vi "Actor Core.vi"(8 "error in":errorcluster, 11 "Manual UI in":refnum<class "Manual UI.lvclass">) -> (0 "error out":errorcluster, 3 "Actor out":refnum<class "Actor.lvclass">)   [LabVIEW 2019, in "Manual UI.lvlib" / "Manual UI.lvclass"]
doc: "The user interface for the main gui panel.\nThis UI manages splitter positions and instrument panels."
uses:
  Project/Manual UI.lvclass
  C:/Users/Public/Documents/Development/builds/Engine/Engine.lvlibp/Project/Engine.lvclass
  builds/Engine/Actor Framework.lvlibp/1abvi3w/vi.lib/ActorFramework/Actor/Actor.lvclass
  Project/Manual UI.lvclass/Manual UI.ctl
  Manual UI Messages/Change Active Instrument Msg/Change Active Instrument Msg.lvclass/Change Active Instrument Msg.ctl
  Accessors/Write instrSplitters.vi
  Accessors/Write instrPanels.vi
  builds/Engine/Engine.lvlibp/Accessors/Write VI_Ref.vi
  builds/Engine/Engine.lvlibp/Accessors/Read Self Q.vi
  builds/Engine/Actor Framework.lvlibp/1abvi3w/vi.lib/ActorFramework/Message Enqueuer/Enqueue.vi
  builds/Engine/Actor Framework.lvlibp/1abvi3w/vi.lib/ActorFramework/Message Enqueuer/Message Enqueuer.lvclass
  Manual UI Messages/Change Active Instrument Msg/Change Active Instrument Msg.lvclass
  Manual UI Messages/Close Instruments Msg/Close Instruments Msg.lvclass
  Manual UI Messages/Launch Instruments Msg/Launch Instruments Msg.lvclass
  builds/Base Software/Panels/Prime Panel.lvlibp/Project/Prime Panel.lvclass
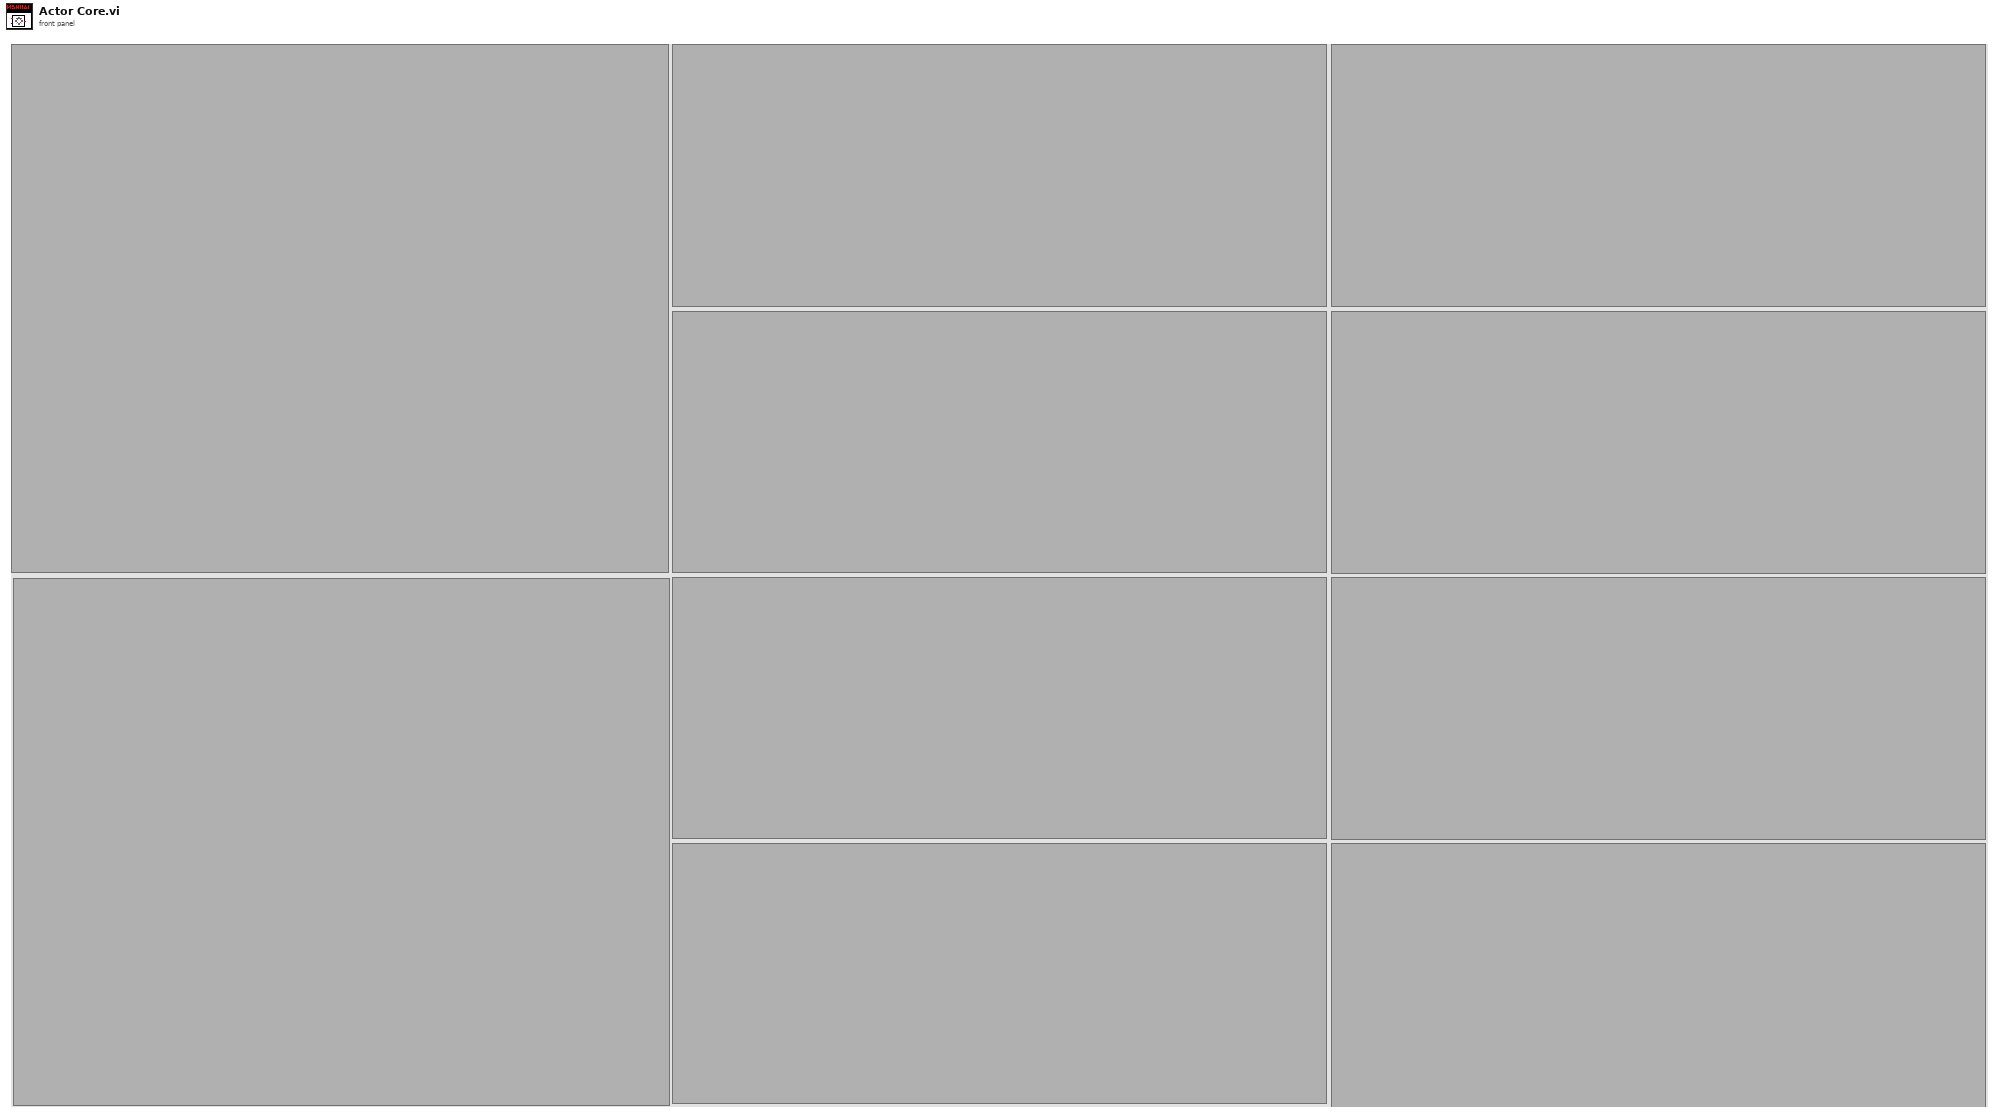
[diagram p1: front panel]
types:
  T1 = cluster{"Pnl Actor":refnum<event-registration>, "Event Registration Refnum":refnum<event-registration>}
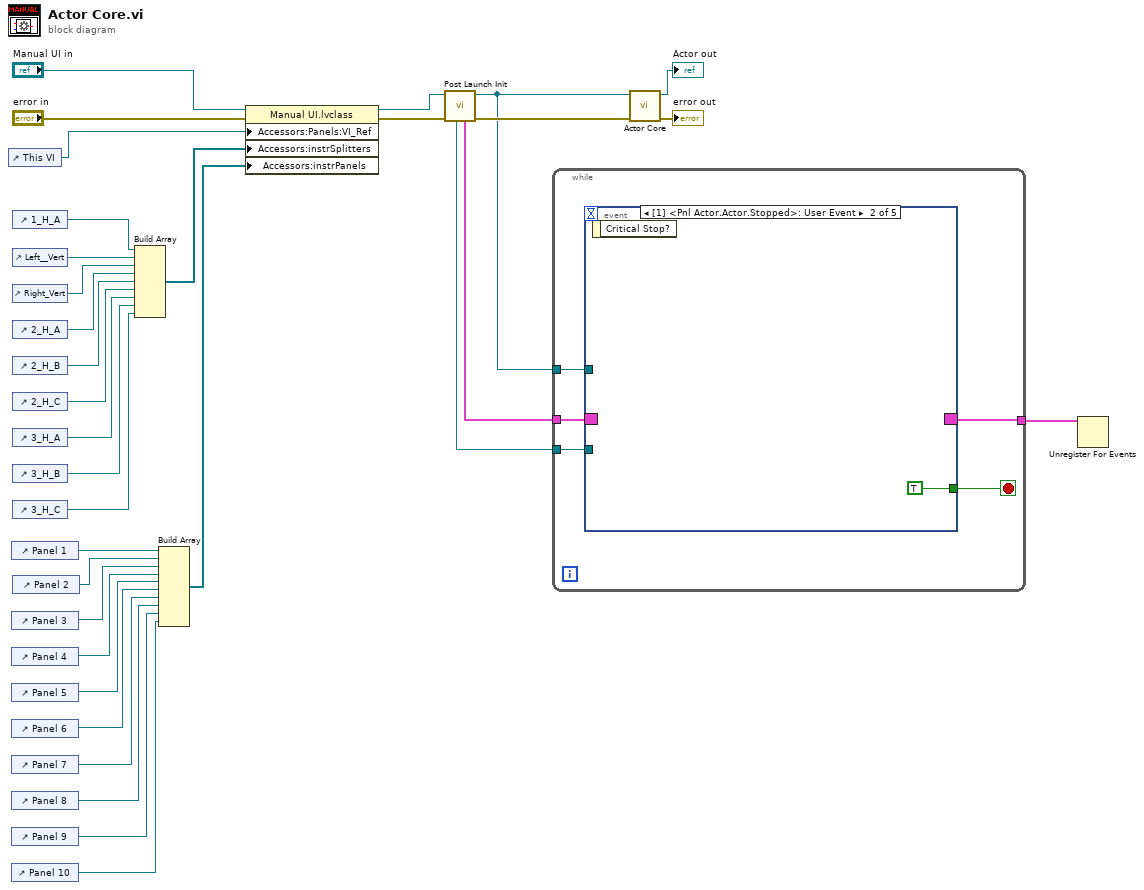
[diagram p0: block diagram]
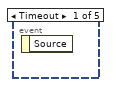
[diagram p2: hidden frame]
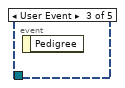
[diagram p3: hidden frame]
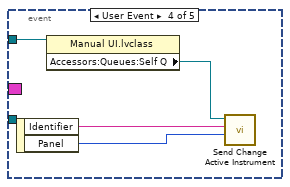
[diagram p4: hidden frame]
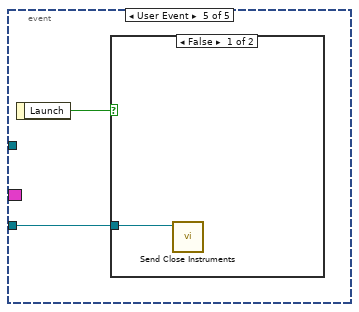
[diagram p5: hidden frame]
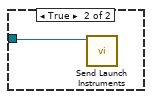
[diagram p6: hidden frame]
diagram:
  n1 = control-ref of="This VI"() -> (w7:refnum<vi>)
  n2 = control-ref of="Panel 1"() -> (w21:refnum<vi>)
  n3 = control-ref of="Panel 3"() -> (w20:refnum<vi>)
  n4 = control-ref of="Panel 4"() -> (w19:refnum<vi>)
  n5 = control-ref of="Panel 5"() -> (w18:refnum<vi>)
  n6 = control-ref of="Panel 6"() -> (w17:refnum<vi>)
  n7 = control-ref of="Panel 7"() -> (w16:refnum<vi>)
  n8 = control-ref of="Panel 8"() -> (w15:refnum<vi>)
  n9 = control-ref of="Panel 9"() -> (w14:refnum<vi>)
  n10 = control-ref of="Panel 10"() -> (w13:refnum<vi>)
  n11 = control-ref of="1_H_A"() -> (w2:refnum<vi>)
  n12 = control-ref of="Left__Vert"() -> (w31:refnum<vi>)
  n13 = control-ref of="Right_Vert"() -> (w30:refnum<vi>)
  n14 = control-ref of="2_H_A"() -> (w29:refnum<vi>)
  n15 = control-ref of="2_H_B"() -> (w28:refnum<vi>)
  n16 = control-ref of="2_H_C"() -> (w27:refnum<vi>)
  n17 = control-ref of="3_H_A"() -> (w26:refnum<vi>)
  n18 = control-ref of="3_H_B"() -> (w25:refnum<vi>)
  n19 = control-ref of="3_H_C"() -> (w24:refnum<vi>)
  n20 = control-ref of="Panel 2"() -> (w1:refnum<vi>)
  n21 = Build Array(w2, w31, w30, w29, w28, w27, w26, w25, w24) -> (w4:refnum<vi>[])
  n22 = Build Array(w21, w1, w20, w19, w18, w17, w16, w15, w14, w13) -> (w12:refnum<vi>[])
  n23 = property class="Manual UI.lvclass"(reference="Manual UI in", error in="error in", "Accessors:Panels:VI_Ref"=w7, "Accessors:instrSplitters"=w4, "Accessors:instrPanels"=w12) -> (reference out=w11:refnum<class "Manual UI.lvclass">, error out=w10:errorcluster)
  n24 = call "Post Launch Init.vi"("error in"=w10, "Manual UI in"=w11) -> ("error out"=w9:errorcluster, "Manual UI out"=w5:refnum<class "Manual UI.lvclass">, "Events"=w8:T1, "Self Enqueuer"=w3:refnum<class "Message Enqueuer.lvclass">)  [unwired: 6 in]
  n25 = while {
    tunnel: w8 -> [w38]
    tunnel: [w36] -> w6
    tunnel: w5 -> [w35]
    tunnel: w3 -> [w34]
    stop <- w37 stop-if-true
    n26 = event shown="[1] <Pnl Actor.Actor.Stopped>: User Event" {
      selector: w38 -> [_ _ _ _ _]
      dyn-events: [_ _ _ _ _] -> w36
      timeout: _ -> [_ _ _ _ _]
      tunnel: [_ TRUE _ _ _] -> w37
      tunnel: w35 -> [_ _ _ w41 _]
      tunnel: w34 -> [_ _ _ _ w44]
      event Timeout {
        n27 = event-data() -> ()  [unwired: 1 in, 1 out]
      }
      event User Event {
        n28 = event-data() -> ()  [unwired: 1 in, 1 out]
      }
      event User Event {
        n29 = event-data() -> ()  [unwired: 1 in, 1 out]
      }
      event User Event {
        n30 = event-data() -> ("Identifier"=w43:string, "Panel"=w42:i32)  [unwired: 1 in]
        n31 = property class="Manual UI.lvclass"(reference=w41) -> ("Accessors:Queues:Self Q"=w40:refnum<class "Message Enqueuer.lvclass">)  [unwired: 1 in, 2 out]
        n32 = call "Send Change Active Instrument.vi"("Panel"=w42, "Identifier"=w43, "Message Enqueuer"=w40) -> ()  [unwired: 7 in, 2 out]
      }
      event User Event {
        n33 = event-data() -> ("Launch"=w45:bool)  [unwired: 1 in]
        n34 = case shown="False" w45 {
          tunnel: w44 -> [w46 w47]
          frame False {
            n35 = call "Send Close Instruments.vi"("Message Enqueuer"=w46) -> ()  [unwired: 9 in, 2 out]
          }
          frame True {
            n36 = call "Send Launch Instruments.vi"("Message Enqueuer"=w47) -> ()  [unwired: 9 in, 2 out]
          }
        }
      }
    }
  }
  n37 = call-parent "Actor Core.vi"("error in"=w9, "Prime Panel in"=w5) -> ("error out"=→"error out":errorcluster, "Actor out"=→"Actor out":refnum<class "Actor.lvclass">)  [unwired: 8 in]
  n38 = Unregister For Events(event registration refnum=w6) -> ()  [unwired: 1 in, 1 out]
